vi "ROS_Master_checkNode.vi"(2 "PubSub":T2, 3 "ROS_Master in":T1) -> (1 "ROS_Master out":T1)   [LabVIEW 2012]
doc: "Checks nodes and closes old nodes"
uses:
  <userlib>/ROSforLV/ROS/Code/ROS_Master/ROS_Topic.ctl
  <userlib>/ROSforLV/ROS/Code/ROS_Master/ROS_Master.ctl
  <userlib>/ROSforLV/ROS/Code/ROS_Master/ROS_Node.ctl
  <userlib>/ROSforLV/ROS/Code/ROS_Master/ROS_Service.ctl
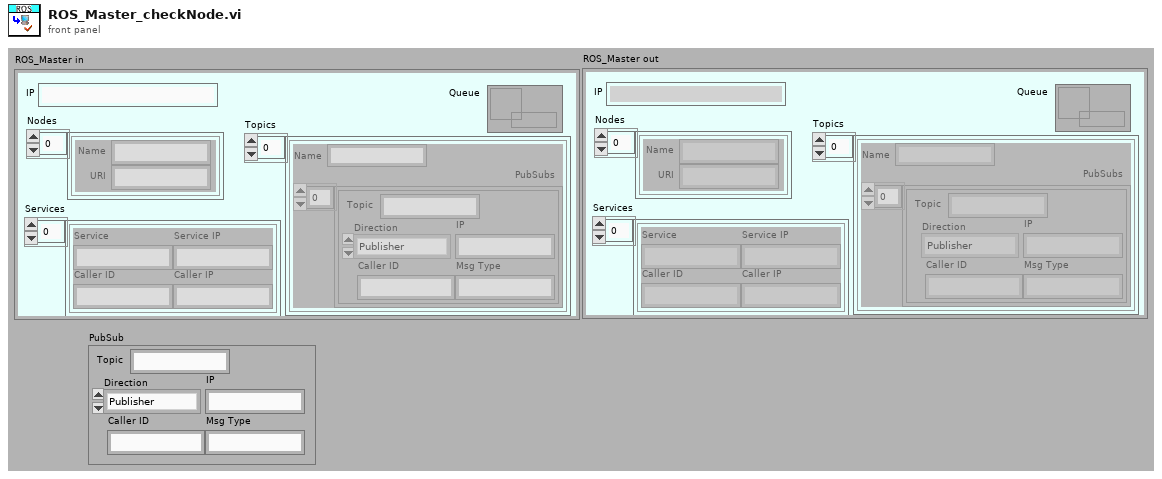
[diagram p1: front panel]
types:
  T1 = typedef "ROS_Master.ctl" = cluster{"IP":string, "Topics":cluster{"Name":string, "PubSubs":T2[]}[], "Nodes":T3[], "Services":T4[], "Queue":refnum<queue>}
  T2 = typedef "ROS_Topic.ctl" = cluster{"Caller ID":string, "IP":string, "Msg Type":string, "Direction":enum16{"Publisher", "Subscriber"}, "Topic":string}
  T3 = typedef "ROS_Node.ctl" = cluster{"Name":string, "URI":string}
  T4 = typedef "ROS_Service.ctl" = cluster{"Service":string, "Service IP":string, "Caller IP":string, "Caller ID":string}
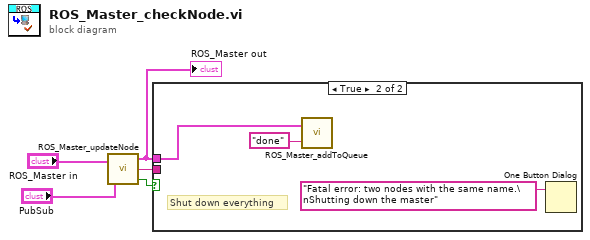
[diagram p0: block diagram]
diagram:
  n1 = call <userlib>:"ROS_Master_updateNode.vi"("ROS_Master in"="ROS_Master in", "PubSub"="PubSub") -> ("ROS_Master in"=w1:T1, "Shutdown URI"=w5:string, "shutdown needed?"=w3:bool)
  "ROS_Master out" <- w1
  n2 = case shown="True" w3 {
    tunnel: w5 -> [_ _]
    tunnel: w1 -> [_ w8]
    frame False {
    }
    frame True {
      # "Shut down everything"
      n3 = call <userlib>:"ROS_Master_addToQueue.vi"("Message"="done" ("format string"), "ROS_Master in"=w8) -> ()  [unwired: 2 in]
      n4 = One Button Dialog(message="Fatal error: two nodes with the same name.\nShutting down the master") -> ()  [unwired: 1 in, 1 out]
    }
  }
